vi "Interfaz.vi"(8 "error in (no error)":errorcluster, 11 "Modulo a obtener":T1=enum."Error") -> (0 "error out":errorcluster)   [LabVIEW 2020]
uses:
  Comunes/Controles/Lista Modulos.ctl
  Comunes/Controles/FGV Opciones.ctl
  Add/Controles e indicadores.ctl
  <vilib>/event_ctls.llb/eventvkey.ctl
  Comunes/Comunicacion/Mensajes.lvlib
panel:
  out "Table":string[][](table)
  in  "Codigo":string
  in  "Agregar":bool
  in  "Vender":bool
  in  "Eliminar":bool
  in  "Aceptar":bool
  in  "Cancelar":bool
  in  "Estadisticas":bool
  in  "Nuevo":bool
  in  "Ver inventario":bool
  in  "Fecha de inicio":timestamp
  in  "Fecha de termino":timestamp
  in  "Color":string(combo)
  in  "Modelo":string(combo)
  in  "Talla":string(combo)
  in  "Buscar":bool
  out "Indicador":string
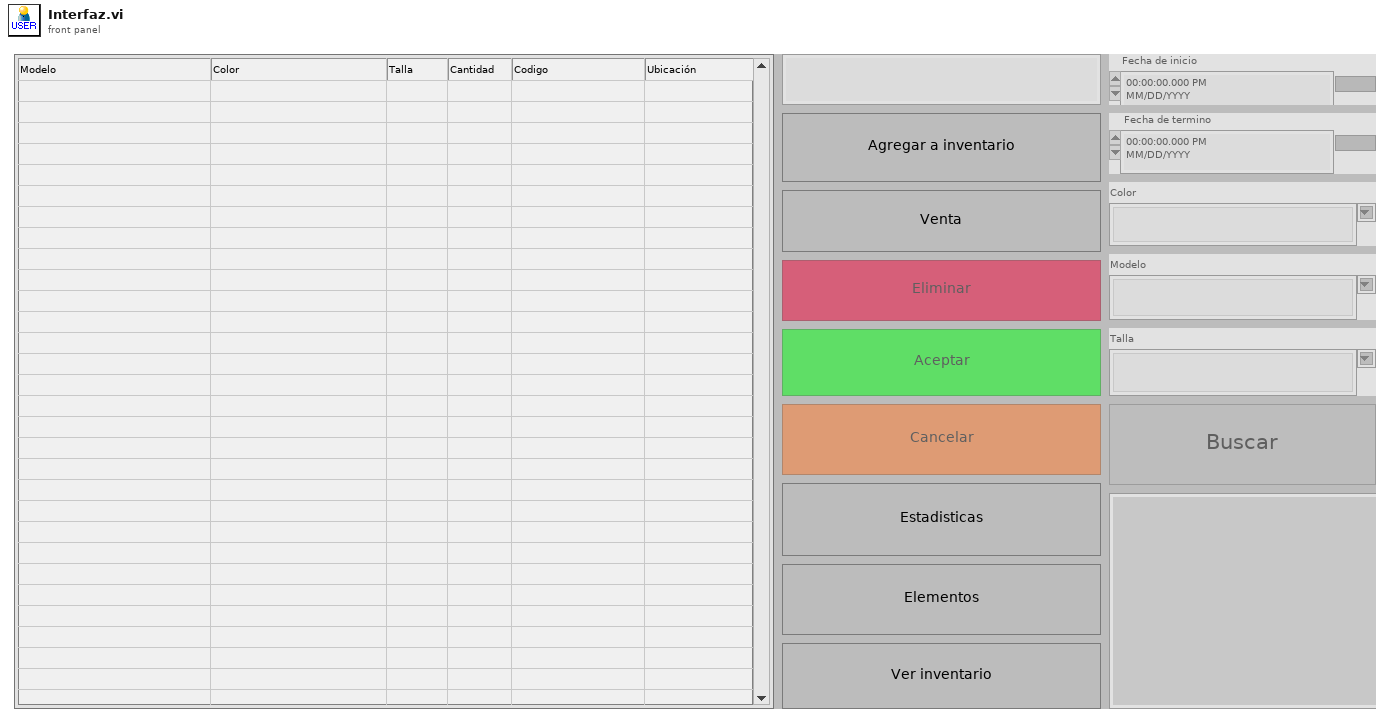
[diagram p1: front panel]
types:
  T1 = typedef "Lista Modulos.ctl" = enum16{"Math", "Error", "Front", "Database", "Nuevos items"}
  T2 = typedef "Controles e indicadores.ctl" = cluster{"Elementos ":refnum<vi>, "Aceptar":refnum<vi>, "Vender":refnum<vi>, "Ver inventario":refnum<vi>, "Agregar":refnum<vi>, "Restar ":refnum<vi>, "Nuevo":refnum<vi>, "Codigo":refnum<vi>, "Grafica":refnum<vi>, "Buscar":refnum<vi>, "Talla":refnum<vi>, "Fecha de termino":refnum<vi>, "Modelo":refnum<vi>, "Fecha de inicio":refnum<vi>, "Color":refnum<vi>, "inventario/ventas":bool, "Eliminar":bool, "Agregar 2":bool, "Vender 2":bool, "Cancelar":refnum<vi>, "Estadisticas":refnum<vi>}
  T3 = typedef "FGV Opciones.ctl" = enum16{"Get", "Create", "Destroy"}
  T4 = enum8{"Enabled", "Disabled", "Disabled and Grayed Out"}
  T5 = enum32{"Invalid", "Standard", "Closed", "Hidden", "Minimized", "Maximized"}
  T6 = typedef "eventvkey.ctl" = enum16{"ASCII", "Enter", "Return", "Shift", "Ctrl", "Alt", "Cmd", "Opt", "Caps", "NumLock", "Clear", "Break", "Up", "Down", "Left", "Right", "Insert", "Delete", "Home", "End", "PageUp", "PageDown", "Escape", "Help", "Pause", "ScrollLock", "F1", "F2", "F3", "F4", "F5", "F6", "F7", "F8", "F9", "F10", "F11", "F12", "F13", "F14", "F15", "F16", "F17", "F18", "F19", "F20", "F21", "F22", "F23", "F24", "Play", "VolumeUp", "VolumeDown", "Mute", "Two Byte Char"}
  T7 = cluster{"Fecha de termino":timestamp, "Fecha de inicio":timestamp, "Modelo":string, "Talla":string, "Color":string}
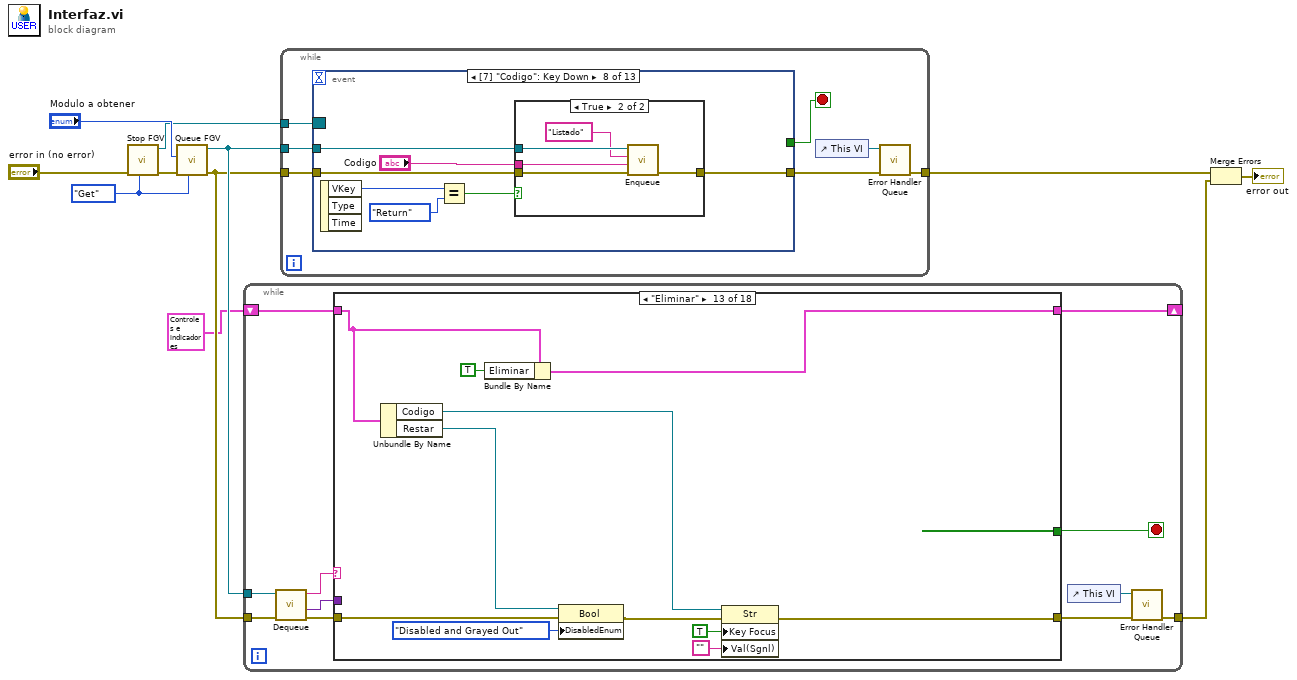
[diagram p0: block diagram]
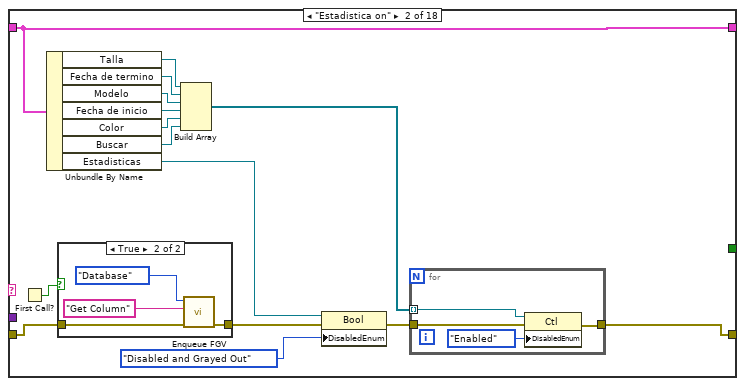
[diagram p3: hidden frame]
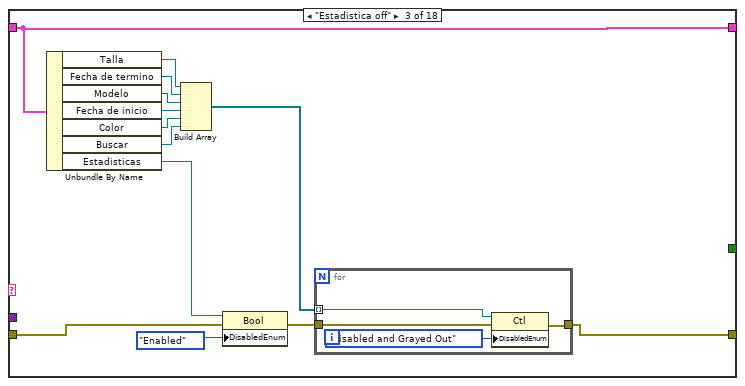
[diagram p5: hidden frame]
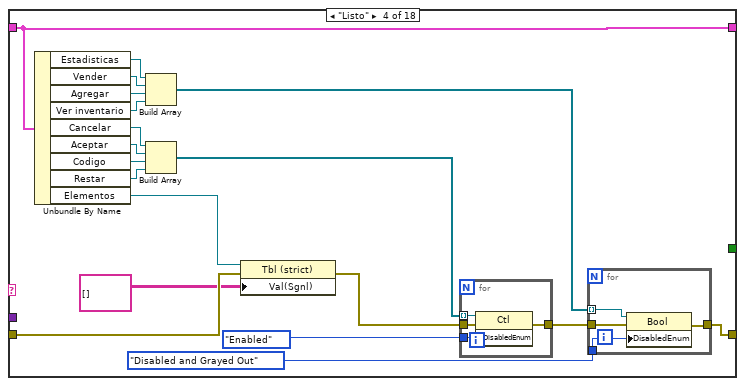
[diagram p6: hidden frame]
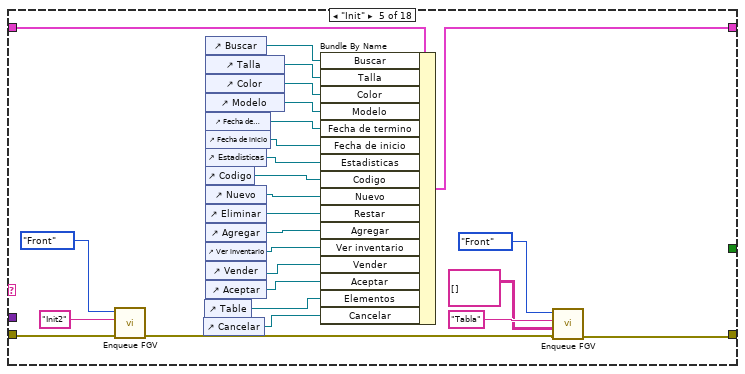
[diagram p7: hidden frame]
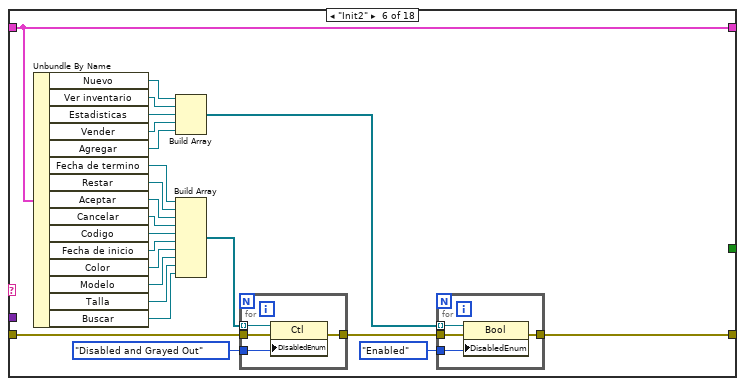
[diagram p8: hidden frame]
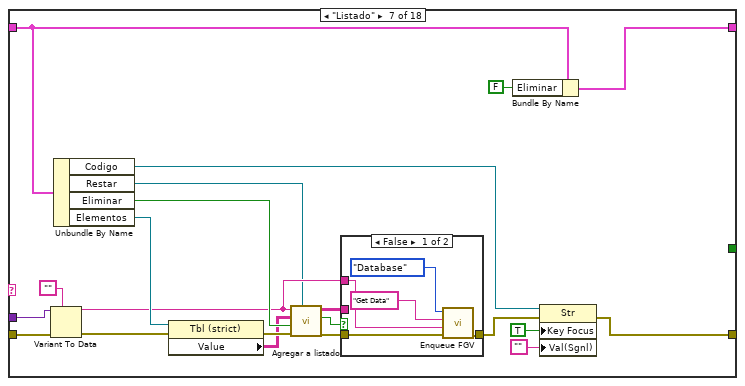
[diagram p9: hidden frame]
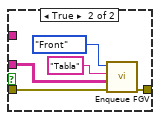
[diagram p10: hidden frame]
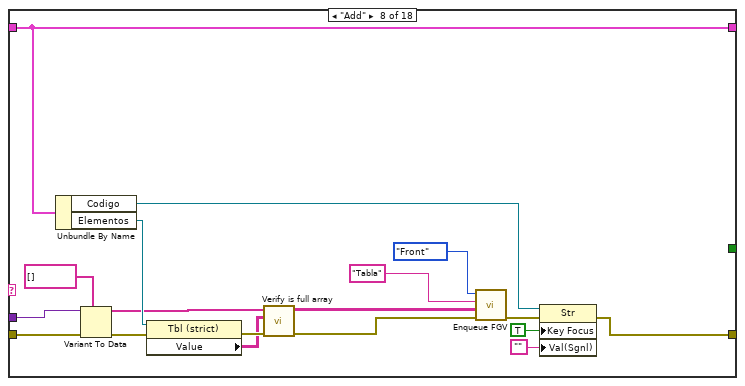
[diagram p11: hidden frame]
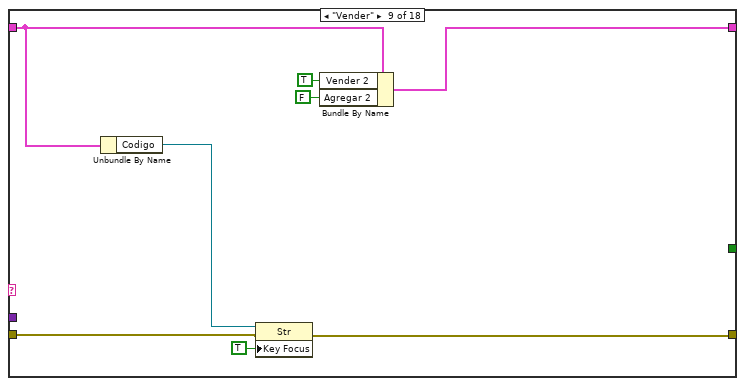
[diagram p12: hidden frame]
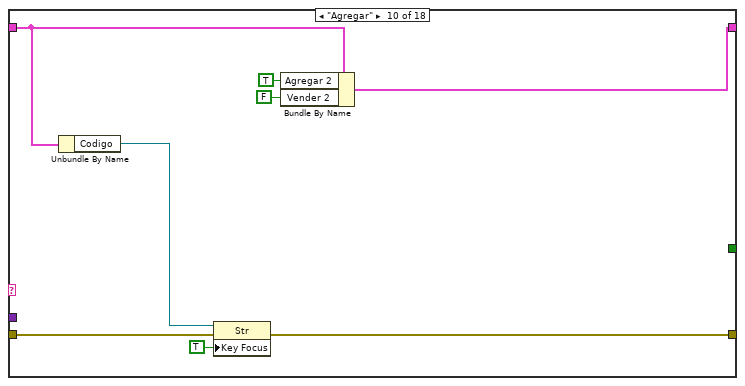
[diagram p13: hidden frame]
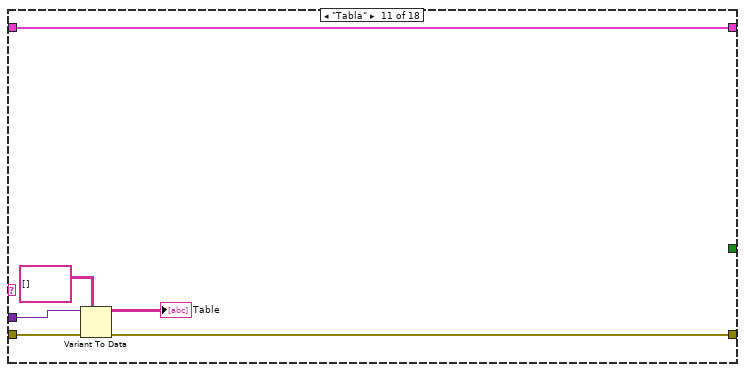
[diagram p14: hidden frame]
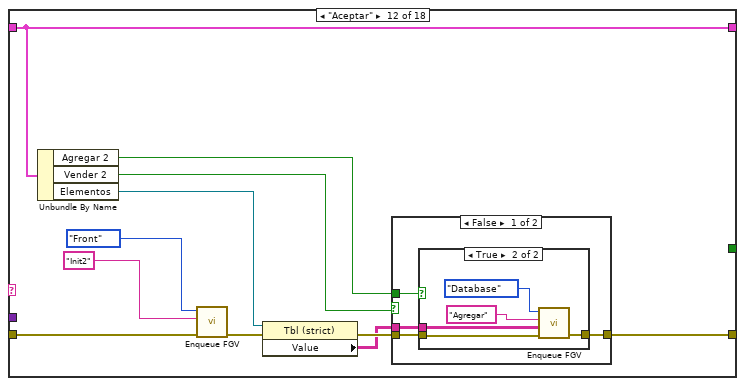
[diagram p15: hidden frame]
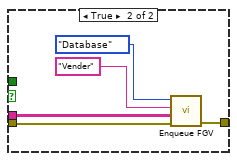
[diagram p17: hidden frame]
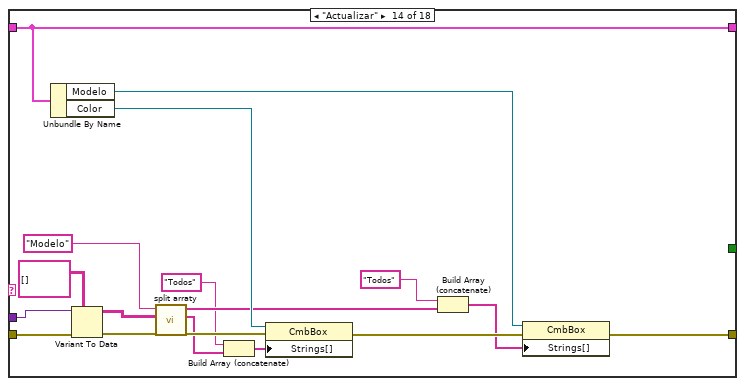
[diagram p18: hidden frame]
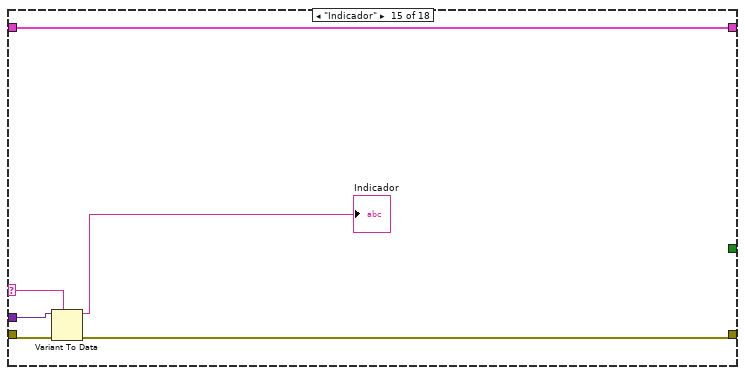
[diagram p19: hidden frame]
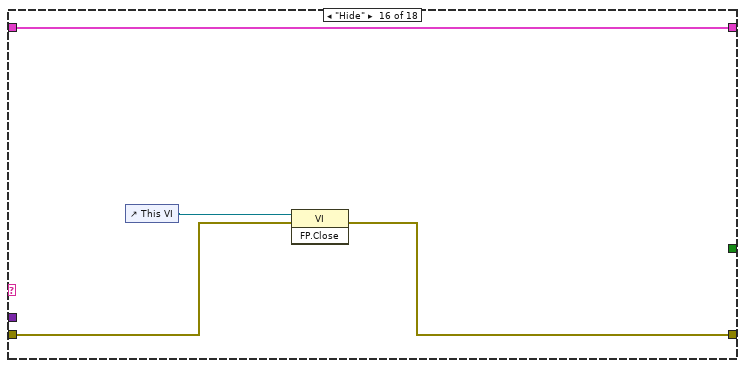
[diagram p20: hidden frame]
diagram:
  w2 = FGV_Opciones."Get" ("Enum")
  n1 = call "Stop FGV.vi"("Enum"=w2, "error in (no error)"="error in (no error)") -> ("error out"=w3:errorcluster, "Event Registration Refnum"=w5:refnum<event-registration>)  [unwired: 7 in, 1 out]
  n2 = call "Queue FGV.vi"("Enum"=w2, "error in (no error)"=w3, "Modulo a obtener"="Modulo a obtener") -> ("error out"=w9:errorcluster, "Queue Ref"=w10:refnum<queue>)  [unwired: 7 in]
  n3 = while {
    tunnel: w10 -> [w22]
    tunnel: w9 -> [w21]
    tunnel: [w15] -> w7
    shift-right: [w13] -> _
    shift-left: T2 {"Elementos "=refnum, "Aceptar"=refnum, "Vender"=refnum, "Ver inventario"=refnum, "Agregar"=refnum, "Restar "=refnum, "Nuevo"=refnum, "Codigo"=refnum, "Grafica"=refnum, "Buscar"=refnum, "Talla"=refnum, "Fecha de termino"=refnum, "Modelo"=refnum, "Fecha de inicio"=refnum, "Color"=refnum, "inventario/ventas"=FALSE, "Eliminar"=FALSE, "Agregar 2"=FALSE, "Vender 2"=FALSE, "Cancelar"=refnum, "Estadisticas"=refnum} ("Cluster") -> [w12]
    stop <- w14 stop-if-true
    n4 = call "Dequeue.vi"("error in (no error)"=w21, "Queue in"=w22) -> ("error out"=w17:errorcluster, "Dato"=w19:variant, "Mensaje"=w20:string)  [unwired: 7 in]
    n5 = case shown="\"Eliminar\"" w20 {
      selector: w20 -> [_ _ _ _ _ _ _ _ _ _ _ _ _ _ w278 _ _ _]
      tunnel: w19 -> [_ _ _ _ _ _ w169 w196 _ _ w218 _ _ w272 w279 _ _ _]
      tunnel: w17 -> [w24 w26 w52 w68 w100 w130 w170 w197 w201 w208 w220 w224 w254 w273 w280 w283 w287 w294]
      tunnel: [w24 w33 w55 w80 w94 w126 w157 w194 w200 w207 w219 w228 w248 w268 w276 w282 w286 w292] -> w16
      tunnel: [_ _ _ _ _ _ _ _ _ _ _ _ _ _ _ _ _ TRUE] -> w14
      tunnel: [w23 w29 w49 w76 w101 w141 w150 w198 w205 w213 w216 w231 w256 w274 w275 w281 w285 w291] -> w13
      tunnel: w12 -> [w23 w29 w49 w76 w118 w141 w152 w198 w199 w211 w216 w231 w255 w274 w275 w281 w285 w291]
      frame "False", Default {
      }
      frame "Estadistica on" {
        n6 = First Call?() -> (First Call?: T/F=w25:bool)
        n7 = Unbundle By Name(w29) -> ("Talla"=w39:refnum<vi>, "Fecha de termino"=w38:refnum<vi>, "Modelo"=w37:refnum<vi>, "Fecha de inicio"=w36:refnum<vi>, "Color"=w35:refnum<vi>, "Buscar"=w34:refnum<vi>, "Estadisticas"=w28:refnum<vi>)
        n8 = case shown="True" w25 {
          tunnel: [w40 w42] -> w27
          tunnel: w26 -> [w40 w41]
          frame False {
          }
          frame True {
            n9 = call "Enqueue FGV.vi"("error in (no error)"=w41, "Mensaje"="Get Column", "Modulo a obtener"=Lista_Modulos."Database") -> ("error out"=w42:errorcluster)  [unwired: 8 in]
          }
        }
        n10 = Build Array(w39, w38, w37, w36, w35, w34) -> (w32:refnum<vi>[])
        n11 = property class="Bool"(reference=w28, error in=w27, "DisabledEnum"=T4."Disabled and Grayed Out" ("Disabled")) -> (error out=w31:errorcluster)  [unwired: 1 out]
        n12 = for {
          tunnel: w32 -> [w46] mode=indexing
          tunnel: w31 -> [w48]
          tunnel: [w47] -> w33
          n13 = property class="Ctl"(reference=w46, error in=w48, "DisabledEnum"=T4."Enabled" ("Disabled")) -> (error out=w47:errorcluster)  [unwired: 1 out]
        }
      }
      frame "Estadistica off" {
        n14 = Unbundle By Name(w49) -> ("Talla"=w61:refnum<vi>, "Fecha de termino"=w60:refnum<vi>, "Modelo"=w59:refnum<vi>, "Fecha de inicio"=w58:refnum<vi>, "Color"=w57:refnum<vi>, "Buscar"=w56:refnum<vi>, "Estadisticas"=w51:refnum<vi>)
        n15 = Build Array(w61, w60, w59, w58, w57, w56) -> (w54:refnum<vi>[])
        n16 = property class="Bool"(reference=w51, error in=w52, "DisabledEnum"=T4."Enabled" ("Disabled")) -> (error out=w53:errorcluster)  [unwired: 1 out]
        n17 = for {
          tunnel: w54 -> [w63] mode=indexing
          tunnel: w53 -> [w65]
          tunnel: [w64] -> w55
          n18 = property class="Ctl"(reference=w63, error in=w65, "DisabledEnum"=T4."Disabled and Grayed Out" ("Disabled")) -> (error out=w64:errorcluster)  [unwired: 1 out]
        }
      }
      frame "Listo" {
        n19 = Unbundle By Name(w76) -> ("Estadisticas"=w84:refnum<vi>, "Vender"=w83:refnum<vi>, "Agregar"=w82:refnum<vi>, "Ver inventario"=w81:refnum<vi>, "Cancelar"=w75:refnum<vi>, "Aceptar"=w74:refnum<vi>, "Codigo"=w73:refnum<vi>, "Restar"=w71:refnum<vi>, "Elementos"=w67:refnum<vi>)
        n20 = Build Array(w84, w83, w82, w81) -> (w79:refnum<vi>[])
        n21 = Build Array(w75, w74, w73, w71) -> (w72:refnum<vi>[])
        n22 = property class="Tbl (strict)"(reference=w67, error in=w68, "Val(Sgnl)"=string[][] [] ("Value (Signaling)")) -> (error out=w69:errorcluster)  [unwired: 1 out]
        n23 = for {
          tunnel: T4."Enabled" ("Disabled") -> [w86]
          tunnel: w69 -> [w87]
          tunnel: [w88] -> w78
          tunnel: w72 -> [w85] mode=indexing
          n24 = property class="Ctl"(reference=w85, error in=w87, "DisabledEnum"=w86) -> (error out=w88:errorcluster)  [unwired: 1 out]
        }
        n25 = for {
          tunnel: w79 -> [w90] mode=indexing
          tunnel: w78 -> [w92]
          tunnel: [w91] -> w80
          tunnel: T4."Disabled and Grayed Out" ("Disabled") -> [w89]
          n26 = property class="Bool"(reference=w90, error in=w92, "DisabledEnum"=w89) -> (error out=w91:errorcluster)  [unwired: 1 out]
        }
      }
      frame "Init" {
        n27 = call "Enqueue FGV.vi"("error in (no error)"=w100, "Mensaje"="Init2", "Modulo a obtener"=Lista_Modulos."Front") -> ("error out"=w95:errorcluster)  [unwired: 8 in]
        n28 = control-ref of="Cancelar"() -> (w102:refnum<vi>)
        n29 = control-ref of="Table"() -> (w109:refnum<vi>)
        n30 = control-ref of="Buscar"() -> (w103:refnum<vi>)
        n31 = control-ref of="Talla"() -> (w104:refnum<vi>)
        n32 = control-ref of="Color"() -> (w105:refnum<vi>)
        n33 = control-ref of="Modelo"() -> (w106:refnum<vi>)
        n34 = control-ref of="Fecha de termino"() -> (w107:refnum<vi>)
        n35 = control-ref of="Fecha de inicio"() -> (w108:refnum<vi>)
        n36 = control-ref of="Estadisticas"() -> (w110:refnum<vi>)
        n37 = control-ref of="Codigo"() -> (w117:refnum<vi>)
        n38 = control-ref of="Nuevo"() -> (w116:refnum<vi>)
        n39 = control-ref of="Eliminar"() -> (w115:refnum<vi>)
        n40 = control-ref of="Agregar"() -> (w114:refnum<vi>)
        n41 = control-ref of="Ver inventario"() -> (w113:refnum<vi>)
        n42 = control-ref of="Vender"() -> (w112:refnum<vi>)
        n43 = control-ref of="Aceptar"() -> (w111:refnum<vi>)
        n44 = Bundle By Name(cluster=w118, "Buscar"=w103, "Talla"=w104, "Color"=w105, "Modelo"=w106, "Fecha de termino"=w107, "Fecha de inicio"=w108, "Estadisticas"=w110, "Codigo"=w117, "Nuevo"=w116, "Restar"=w115, "Agregar"=w114, "Ver inventario"=w113, "Vender"=w112, "Aceptar"=w111, "Elementos"=w109, "Cancelar"=w102) -> (w101:T2)
        n45 = call "Enqueue FGV.vi"("error in (no error)"=w95, "Dato"=string[][] [] ("type"), "Mensaje"="Tabla", "Modulo a obtener"=Lista_Modulos."Front") -> ("error out"=w94:errorcluster)  [unwired: 7 in]
      }
      frame "Init2" {
        n46 = Unbundle By Name(w141) -> ("Nuevo"=w125:refnum<vi>, "Ver inventario"=w124:refnum<vi>, "Estadisticas"=w123:refnum<vi>, "Vender"=w122:refnum<vi>, "Agregar"=w121:refnum<vi>, "Fecha de termino"=w140:refnum<vi>, "Restar"=w139:refnum<vi>, "Aceptar"=w138:refnum<vi>, "Cancelar"=w137:refnum<vi>, "Codigo"=w136:refnum<vi>, "Fecha de inicio"=w135:refnum<vi>, "Color"=w134:refnum<vi>, "Modelo"=w133:refnum<vi>, "Talla"=w132:refnum<vi>, "Buscar"=w131:refnum<vi>)
        n47 = Build Array(w125, w124, w123, w122, w121) -> (w120:refnum<vi>[])
        n48 = Build Array(w140, w139, w138, w137, w136, w135, w134, w133, w132, w131) -> (w129:refnum<vi>[])
        n49 = for {
          tunnel: w130 -> [w149]
          tunnel: [w148] -> w127
          tunnel: w129 -> [w147] mode=indexing
          tunnel: T4."Disabled and Grayed Out" ("Disabled") -> [w146]
          n50 = property class="Ctl"(reference=w147, error in=w149, "DisabledEnum"=w146) -> (error out=w148:errorcluster)  [unwired: 1 out]
        }
        n51 = for {
          tunnel: w127 -> [w145]
          tunnel: [w144] -> w126
          tunnel: w120 -> [w143] mode=indexing
          tunnel: T4."Enabled" ("Disabled") -> [w142]
          n52 = property class="Bool"(reference=w143, error in=w145, "DisabledEnum"=w142) -> (error out=w144:errorcluster)  [unwired: 1 out]
        }
      }
      frame "Listado" {
        n53 = Variant To Data(error in=w170, type="", Variant=w169) -> (data=w161:string, error out=w159:errorcluster)
        n54 = Unbundle By Name(w152) -> ("Codigo"=w153:refnum<vi>, "Restar"=w154:refnum<vi>, "Eliminar"=w165:bool, "Elementos"=w167:refnum<vi>)
        n55 = property class="Tbl (strict)"(reference=w167, error in=w159) -> (error out=w166:errorcluster, "Value"=w164:string[][])  [unwired: 1 out]
        n56 = call "Agregar a listado.vi"("Restar"=w154, "error in (no error)"=w166, "Restar?"=w165, "Listado"=w164, "Codigo"=w161) -> ("error out"=w163:errorcluster, "Encontrado?"=w162:bool, "Listado 2"=w160:string[][])  [unwired: 4 in]
        n57 = case shown="False" w162 {
          tunnel: [w174 w180] -> w158
          tunnel: w163 -> [w175 w179]
          tunnel: w161 -> [w172 _]
          tunnel: w160 -> [_ w178]
          frame False {
            n58 = call "Enqueue FGV.vi"("error in (no error)"=w175, "Dato"=w172, "Mensaje"="Get Data", "Modulo a obtener"=Lista_Modulos."Database") -> ("error out"=w174:errorcluster)  [unwired: 7 in]
          }
          frame True {
            n59 = call "Enqueue FGV.vi"("error in (no error)"=w179, "Dato"=w178, "Mensaje"="Tabla", "Modulo a obtener"=Lista_Modulos."Front") -> ("error out"=w180:errorcluster)  [unwired: 7 in]
          }
        }
        n60 = Bundle By Name(cluster=w152, "Eliminar"=FALSE) -> (w150:T2)
        n61 = property class="Str"(reference=w153, error in=w158, "Key Focus"=TRUE, "Val(Sgnl)"="") -> (error out=w157:errorcluster)  [unwired: 1 out]
      }
      frame "Add" {
        n62 = Unbundle By Name(w198) -> ("Codigo"=w186:refnum<vi>, "Elementos"=w195:refnum<vi>)
        n63 = Variant To Data(error in=w197, type=string[] [], Variant=w196) -> (data=w190:string[], error out=w185:errorcluster)
        n64 = property class="Tbl (strict)"(reference=w195, error in=w185) -> (error out=w184:errorcluster, "Value"=w182:string[][])  [unwired: 1 out]
        n65 = call "Verify is full array.vi"("error in (no error)"=w184, "Value"=w182, "Array in"=w190) -> ("error out"=w183:errorcluster, "Data Salida"=w181:string[][])  [unwired: 7 in]
        n66 = call "Enqueue FGV.vi"("error in (no error)"=w183, "Dato"=w181, "Mensaje"="Tabla", "Modulo a obtener"=Lista_Modulos."Front") -> ("error out"=w189:errorcluster)  [unwired: 7 in]
        n67 = property class="Str"(reference=w186, error in=w189, "Key Focus"=TRUE, "Val(Sgnl)"="") -> (error out=w194:errorcluster)  [unwired: 1 out]
      }
      frame "Vender" {
        n68 = Unbundle By Name(w199) -> ("Codigo"=w203:refnum<vi>)
        n69 = property class="Str"(reference=w203, error in=w201, "Key Focus"=TRUE) -> (error out=w200:errorcluster)  [unwired: 1 out]
        n70 = Bundle By Name(cluster=w199, "Vender 2"=TRUE, "Agregar 2"=FALSE) -> (w205:T2)
      }
      frame "Agregar" {
        n71 = Unbundle By Name(w211) -> ("Codigo"=w210:refnum<vi>)
        n72 = property class="Str"(reference=w210, error in=w208, "Key Focus"=TRUE) -> (error out=w207:errorcluster)  [unwired: 1 out]
        n73 = Bundle By Name(cluster=w211, "Agregar 2"=TRUE ("Vender 2"), "Vender 2"=FALSE) -> (w213:T2)
      }
      frame "Tabla" {
        n74 = Variant To Data(error in=w220, type=string[][] [], Variant=w218) -> (data=→"Table":string[][], error out=w219:errorcluster)
      }
      frame "Aceptar" {
        n75 = Unbundle By Name(w231) -> ("Agregar 2"=w225:bool, "Vender 2"=w227:bool, "Elementos"=w230:refnum<vi>)
        n76 = call "Enqueue FGV.vi"("error in (no error)"=w224, "Mensaje"="Init2", "Modulo a obtener"=Lista_Modulos."Front") -> ("error out"=w223:errorcluster)  [unwired: 8 in]
        n77 = property class="Tbl (strict)"(reference=w230, error in=w223) -> (error out=w229:errorcluster, "Value"=w226:string[][])  [unwired: 1 out]
        n78 = case shown="False" w227 {
          tunnel: w229 -> [w235 w245]
          tunnel: [w234 w246] -> w228
          tunnel: w226 -> [w233 w243]
          tunnel: w225 -> [w232 _]
          frame False {
            n79 = case shown="True" w232 {
              tunnel: w235 -> [w236 w240]
              tunnel: [w236 w241] -> w234
              tunnel: w233 -> [_ w239]
              frame False {
              }
              frame True {
                n80 = call "Enqueue FGV.vi"("error in (no error)"=w240, "Dato"=w239, "Mensaje"="Agregar", "Modulo a obtener"=Lista_Modulos."Database") -> ("error out"=w241:errorcluster)  [unwired: 7 in]
              }
            }
          }
          frame True {
            n81 = call "Enqueue FGV.vi"("error in (no error)"=w245, "Dato"=w243, "Mensaje"="Vender", "Modulo a obtener"=Lista_Modulos."Database") -> ("error out"=w246:errorcluster)  [unwired: 7 in]
          }
        }
      }
      frame "Eliminar" {
        n82 = Unbundle By Name(w255) -> ("Codigo"=w247:refnum<vi>, "Restar"=w253:refnum<vi>)
        n83 = Bundle By Name(cluster=w255, "Eliminar"=TRUE) -> (w256:T2)
        n84 = property class="Bool"(reference=w253, error in=w254, "DisabledEnum"=T4."Disabled and Grayed Out" ("Disabled")) -> (error out=w249:errorcluster)  [unwired: 1 out]
        n85 = property class="Str"(reference=w247, error in=w249, "Key Focus"=TRUE, "Val(Sgnl)"="") -> (error out=w248:errorcluster)  [unwired: 1 out]
      }
      frame "Actualizar" {
        n86 = Unbundle By Name(w274) -> ("Modelo"=w264:refnum<vi>, "Color"=w265:refnum<vi>)
        n87 = Variant To Data(error in=w273, type=string[][] [], Variant=w272) -> (data=w271:string[][], error out=w266:errorcluster)
        n88 = call "split arraty.vi"("Datos bruto"=w271, "Parametro"="Modelo") -> ("Datos segundo parametro"=w258:string[], "Datos parametro"=w262:string[])  [unwired: 8 in]
        n89 = Build Array (concatenate)("Todos" ("Parametro"), w258) -> (w259:string[])
        n90 = property class="CmbBox"(reference=w265, error in=w266, "Strings[]"=w259) -> (error out=w267:errorcluster)  [unwired: 1 out]
        n91 = Build Array (concatenate)("Todos" ("Parametro"), w262) -> (w263:string[])
        n92 = property class="CmbBox"(reference=w264, error in=w267, "Strings[]"=w263) -> (error out=w268:errorcluster)  [unwired: 1 out]
      }
      frame "Indicador" {
        n93 = Variant To Data(error in=w280, type=w278, Variant=w279) -> (data=→"Indicador":string, error out=w276:errorcluster)
      }
      frame "Hide" {
        n94 = control-ref of="This VI"() -> (w284:refnum<vi>)
        n95 = invoke class="VI" method="FP.Close"(reference=w284, error in=w283) -> (error out=w282:errorcluster)  [unwired: 1 in, 2 out]
      }
      frame "Show" {
        n96 = control-ref of="This VI"() -> (w288:refnum<vi>)
        n97 = invoke class="VI" method="FP.Open"(reference=w288, error in=w287, "Activate"=TRUE ("Activate?"), "State"=T5."Standard") -> (error out=w286:errorcluster)  [unwired: 1 in, 4 out]
      }
      frame "Stop" {
        n98 = call "Fire Stop.vi"("error in (no error)"=w294) -> ("error out"=w292:errorcluster)  [unwired: 10 in]
      }
    }
    n99 = control-ref of="This VI"() -> (w18:refnum<vi>)
    n100 = call "Error Handler Queue.vi"("error in (no error)"=w16, "VI Refnum"=w18) -> ("error out"=w15:errorcluster)  [unwired: 9 in]
  }
  n101 = while {
    tunnel: w10 -> [w301]
    tunnel: w9 -> [w300]
    tunnel: [w298] -> w8
    tunnel: w5 -> [w296]
    stop <- w295 stop-if-true
    n102 = event shown="[7] \"Codigo\": Key Down" {
      selector: w296 -> [_ _ _ _ _ _ _ _ _ _ _ _ _]
      dyn-events: _ -> [_ _ _ _ _ _ _ _ _ _ _ _ _]
      timeout: _ -> [_ _ _ _ _ _ _ _ _ _ _ _ _]
      tunnel: w301 -> [w304 w307 w313 w318 _ w328 w340 w344 w358 w361 w365 w369 w374]
      tunnel: w300 -> [w303 w308 w312 w319 w325 w329 w332 w345 w359 w363 w367 w373 w378]
      tunnel: [w302 w305 w310 w321 w322 w327 w341 w343 w356 w362 w366 w370 w376] -> w297
      tunnel: [_ TRUE _ _ _ _ _ _ _ _ _ _ _] -> w295
      event Timeout {
        n103 = event-data() -> ()  [unwired: 1 in, 3 out]
        n104 = call "Enqueue.vi"("error in (no error)"=w303, "Queue in"=w304) -> ("error out"=w302:errorcluster)  [unwired: 9 in]
      }
      event User Event {
        n105 = event-data() -> ()  [unwired: 1 in, 3 out]
        n106 = call "Enqueue.vi"("error in (no error)"=w308, "Mensaje"="Stop", "Queue in"=w307) -> ("error out"=w305:errorcluster)  [unwired: 8 in]
      }
      event Panel Close? {
        n107 = event-data() -> ()  [unwired: 1 in, 3 out]
        n108 = call "Enqueue.vi"("error in (no error)"=w312, "Mensaje"="Stop", "Queue in"=w313) -> ("error out"=w310:errorcluster)  [unwired: 8 in]
        n109 = event-data("Discard?"=TRUE) -> ()  [unwired: 1 in, 1 out]
      }
      event "Nuevo": Value Change {
        n110 = event-data() -> ()  [unwired: 1 in, 3 out]
        n111 = call "Enqueue.vi"("error in (no error)"=w319, "Mensaje"="Hide", "Queue in"=w318) -> ("error out"=w320:errorcluster)  [unwired: 8 in]
        n112 = call "Enqueue FGV.vi"("error in (no error)"=w320, "Mensaje"="Show", "Modulo a obtener"=Lista_Modulos."Nuevos items") -> ("error out"=w321:errorcluster)  [unwired: 8 in]
      }
      event "Ver inventario": Value Change {
        n113 = event-data() -> ()  [unwired: 1 in, 3 out]
        n114 = call "Enqueue FGV.vi"("error in (no error)"=w325, "Mensaje"="Ver", "Modulo a obtener"=Lista_Modulos."Database") -> ("error out"=w322:errorcluster)  [unwired: 8 in]
      }
      event "Estadisticas": Value Change {
        n115 = event-data() -> ()  [unwired: 1 in, 3 out]
        n116 = call "Enqueue.vi"("error in (no error)"=w329, "Mensaje"="Estadistica on", "Queue in"=w328) -> ("error out"=w327:errorcluster)  [unwired: 8 in]
      }
      event "Buscar": Value Change {
        n117 = event-data() -> ()  [unwired: 1 in, 3 out]
        n118 = Bundle("Fecha de termino"="Fecha de termino", "Fecha de inicio"="Fecha de inicio", "Modelo"="Modelo", "Talla"="Talla", "Color"="Color") -> (w331:T7)  [unwired: 1 in]
        n119 = call "Enqueue FGV.vi"("error in (no error)"=w332, "Dato"=w331, "Mensaje"="Estadistica", "Modulo a obtener"=Lista_Modulos."Database") -> ("error out"=w334:errorcluster)  [unwired: 7 in]
        n120 = call "Enqueue.vi"("error in (no error)"=w334, "Mensaje"="Estadistica off", "Queue in"=w340) -> ("error out"=w341:errorcluster)  [unwired: 8 in]
      }
      event "Codigo": Key Down {
        n121 = event-data() -> ("VKey"=w346:T6)  [unwired: 1 in, 2 out]
        n122 = Equal?(x=w346, y=eventvkey."Return" ("VKey")) -> (x = y?=w348:bool)
        n123 = case shown="True" w348 {
          tunnel: "Codigo" -> [_ w353]
          tunnel: w345 -> [w350 w355]
          tunnel: w344 -> [_ w354]
          tunnel: [w350 w352] -> w343
          frame False {
          }
          frame True {
            n124 = call "Enqueue.vi"("error in (no error)"=w355, "Dato"=w353, "Mensaje"="Listado", "Queue in"=w354) -> ("error out"=w352:errorcluster)  [unwired: 7 in]
          }
        }
      }
      event "Eliminar": Value Change {
        n125 = event-data() -> ()  [unwired: 1 in, 3 out]
        n126 = call "Enqueue.vi"("error in (no error)"=w359, "Mensaje"="Eliminar", "Queue in"=w358) -> ("error out"=w356:errorcluster)  [unwired: 8 in]
      }
      event "Cancelar": Value Change {
        n127 = event-data() -> ()  [unwired: 1 in, 3 out]
        n128 = call "Enqueue.vi"("error in (no error)"=w363, "Mensaje"="Init2", "Queue in"=w361) -> ("error out"=w362:errorcluster)  [unwired: 8 in]
      }
      event "Aceptar": Value Change {
        n129 = event-data() -> ()  [unwired: 1 in, 3 out]
        n130 = call "Enqueue.vi"("error in (no error)"=w367, "Mensaje"="Aceptar", "Queue in"=w365) -> ("error out"=w366:errorcluster)  [unwired: 8 in]
      }
      event "Agregar": Value Change {
        n131 = event-data() -> ()  [unwired: 1 in, 3 out]
        n132 = call "Enqueue.vi"("error in (no error)"=w373, "Mensaje"="Agregar", "Queue in"=w369) -> ("error out"=w371:errorcluster)  [unwired: 8 in]
        n133 = call "Enqueue.vi"("error in (no error)"=w371, "Mensaje"="Listo", "Queue in"=w369) -> ("error out"=w370:errorcluster)  [unwired: 8 in]
      }
      event "Vender": Value Change {
        n134 = event-data() -> ()  [unwired: 1 in, 3 out]
        n135 = call "Enqueue.vi"("error in (no error)"=w378, "Mensaje"="Vender", "Queue in"=w374) -> ("error out"=w377:errorcluster)  [unwired: 8 in]
        n136 = call "Enqueue.vi"("error in (no error)"=w377, "Mensaje"="Listo", "Queue in"=w374) -> ("error out"=w376:errorcluster)  [unwired: 8 in]
      }
    }
    n137 = control-ref of="This VI"() -> (w299:refnum<vi>)
    n138 = call "Error Handler Queue.vi"("error in (no error)"=w297, "VI Refnum"=w299) -> ("error out"=w298:errorcluster)  [unwired: 9 in]
  }
  n139 = Merge Errors(w8, w7) -> (→"error out":errorcluster)
